vi "PXIe-7962_FPGA.vi"() -> ()   [LabVIEW 2014]
uses:
  <instrlib>/_niInstr/Streaming/v1/Common/Stream State.ctl
  <vilib>/Platform/TimedLoop/XDataNode/timing_clust.ctl
  <vilib>/Platform/TimedLoop/XDataNode/nitl_modes.ctl
  <vilib>/Platform/TimedLoop/XDataNode/wakeup.ctl
  FPGA_Controls/Acquisition FIFOs Cluster.ctl
  <vilib>/rvi/Emulation/niFpgaSctlEmulationGetInTimedLoop.vi
  <vilib>/rvi/Emulation/niFpgaEmulationReportErrorSimple.vi
  <vilib>/rvi/Emulation/niFpgaGetClockAttributes.vi
  <vilib>/rvi/Emulation/niFpgaCriticalErrorInLSC.vi
  <vilib>/rvi/eio/common/nirviEmuTemplateMethod_errors.vi
  <vilib>/rvi/interface/RandomDataEmulation/niFpgaRandomDataHandleErrors.vi
  <vilib>/rvi/DataTransferAndStorage/Container/Common/niFpgaContainerExecOnDevCompGetState.vi
  <vilib>/rvi/Emulation/niFpgaEmulationIsFPGAContextNoSignature.vi
  <vilib>/rvi/errors/niFpgaSetErrorForExecOnDevCompSimple.vi
  <vilib>/rvi/eio/common/nirviEmuReportErrorAndStop.vi
  <vilib>/rvi/DataTransferAndStorage/Container/Common/niFpgaContainerGetUniqueNameForEmu.vi
  <vilib>/rvi/FIFO/Fifo_Resource/nirvififoEmulationSetSize.vi
  <vilib>/rvi/FIFO/Fifo_Resource/nirviFifoEmulationQueueMgr.vi
  <instcachedir>/0/nirviFifoEmulationQueueMgr_E5CAEC123FF24DC58D834DCA3CDAA9B5.lvgen/nirviFifoEmulationQueueMgr_E5CAEC123FF24DC58D834DCA3CDAA9B5_004.vi
  <vilib>/rvi/FIFO/Fifo_Resource/nirvififoEmulationDetermineInputValidOut.vi
  <vilib>/rvi/FIFO/Fifo_Resource/nirvififoEmulationCreateLock.vi
  <vilib>/rvi/Emulation/niFpgaProcessEmulError.vi
  <vilib>/rvi/FIFO/Fifo_Resource/nirvififoEmulationObtainLock.vi
  <vilib>/rvi/FIFO/Fifo_Resource/nirvififoEmulationReleaseLock.vi
  <vilib>/rvi/occurrence/nirviWaitOnOccurrenceBase.vi
  <vilib>/rvi/errors/nirviReportUnexpectedCaseInternalError.vi
  <vilib>/rvi/errors/nirviReportUnexpectedCaseInternalError (U32).vi
  <vilib>/Utility/error.llb/Clear Errors.vi
  <instcachedir>/0/nirviFifoEmulationQueueMgr_E5CAEC123FF24DC58D834DCA3CDAA9B5.lvgen/nirviFifoEmulationQueueMgr_E5CAEC123FF24DC58D834DCA3CDAA9B5_003.vi
  <vilib>/Platform/TimedLoop/XDataNode/XDataNode.xnode
  <vilib>/eio/EIONode/EIONode.xnode
  <vilib>/rvi/DataTransferAndStorage/Container/XNode/niFpgaContainer.xnode
  <vilib>/rvi/interface/RandomDataEmulation/nirviRandomDataFpgaReadWriteTemplate.vi
  <vilib>/rvi/FIFO/Fifo_Resource/niFpgaFifoEmulationRefIn.vi
  <vilib>/rvi/FIFO/Fifo_Resource/nirvififoEmulationWrite.vi
  <vilib>/Platform/TimedLoop/XDataNode/XDNodeRunTimeDep.lvlib
  <instrlib>/_niInstr/Streaming/v1/FPGA/niInstr Streaming v1 FPGA.lvlib
  <instrlib>/_niInstr/Streaming/v1/Common/niInstr Streaming v1 Common.lvlib
panel:
  out "Init Done":bool
  in  "stream.num samples 1":u64
  out "stream.state 1":T1
  out "stream.samples transferred 1":u64
  in  "stream.request state 1":T1
  out "stream.metadata 1":u64
  out "stream.metadata 0":u64
  in  "stream.request state 0":T1
  out "stream.samples transferred 0":u64
  out "stream.state 0":T1
  in  "stream.num samples 0":u64
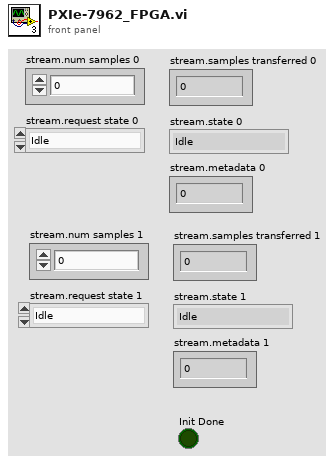
[diagram p1: front panel]
types:
  T1 = typedef "niInstr Streaming v1 Common.lvlib/Stream State.ctl" = enum8{"Idle", "Finite Transfer", "Continuous", "Done", "Error", "Not Ready", "Cancel"}
  T2 = typedef "XDNodeRunTimeDep.lvlib/timing_clust.ctl" = cluster{"Expected End [f-1]":u64, "Actual End [f-1]":u64, "Finished Late? [f-1]":bool, "Expected End [i-1]":u64, "Actual End [i-1]":u64, "Finished Late? [i-1]":bool, "Expected Start [i]":u64, "Actual Start [i]":u64, "Expected Start [f]":u64, "Actual Start [f]":u64, "Source Name":string, "Structure Name":string, "Period":i64, "Deadline":i64, "Offset":i64, "Start":i64, "Priority":i32, "Timeout":i32, "Mode":T3, "Wakeup Reason":T4, "Error":errorcluster, "Source Type":string, "Secondary Source Type":string, "Global End Time":u64, "Global Start Time":u64, "Frame Duration":u64, "Iteration Duration":u64, "Assigned CPU":i32, "I/O Scan Engine Mode":u32}
  T3 = typedef "XDNodeRunTimeDep.lvlib/nitl_modes.ctl" = enum32{"No Change", "Process missed periods, maintain original phase", "Discard missed periods, maintain original phase", "Process missed periods, ignore original phase", "Discard missed periods, ignore original phase"}
  T4 = typedef "XDNodeRunTimeDep.lvlib/wakeup.ctl" = enum32{"Normal", "Aborted", "Asynchronous wakeup", "Timing source error", "Timed loop error", "Timeout"}
  T5 = typedef "Acquisition FIFOs Cluster.ctl" = cluster{"FIFO 0":refnum<k21>, "FIFO 1":refnum<k21>, "FIFO 2":refnum<k21>, "FIFO 3":refnum<k21>, "FIFO 4":refnum<k21>, "FIFO 5":refnum<k21>, "FIFO 6":refnum<k21>, "FIFO 7":refnum<k21>}
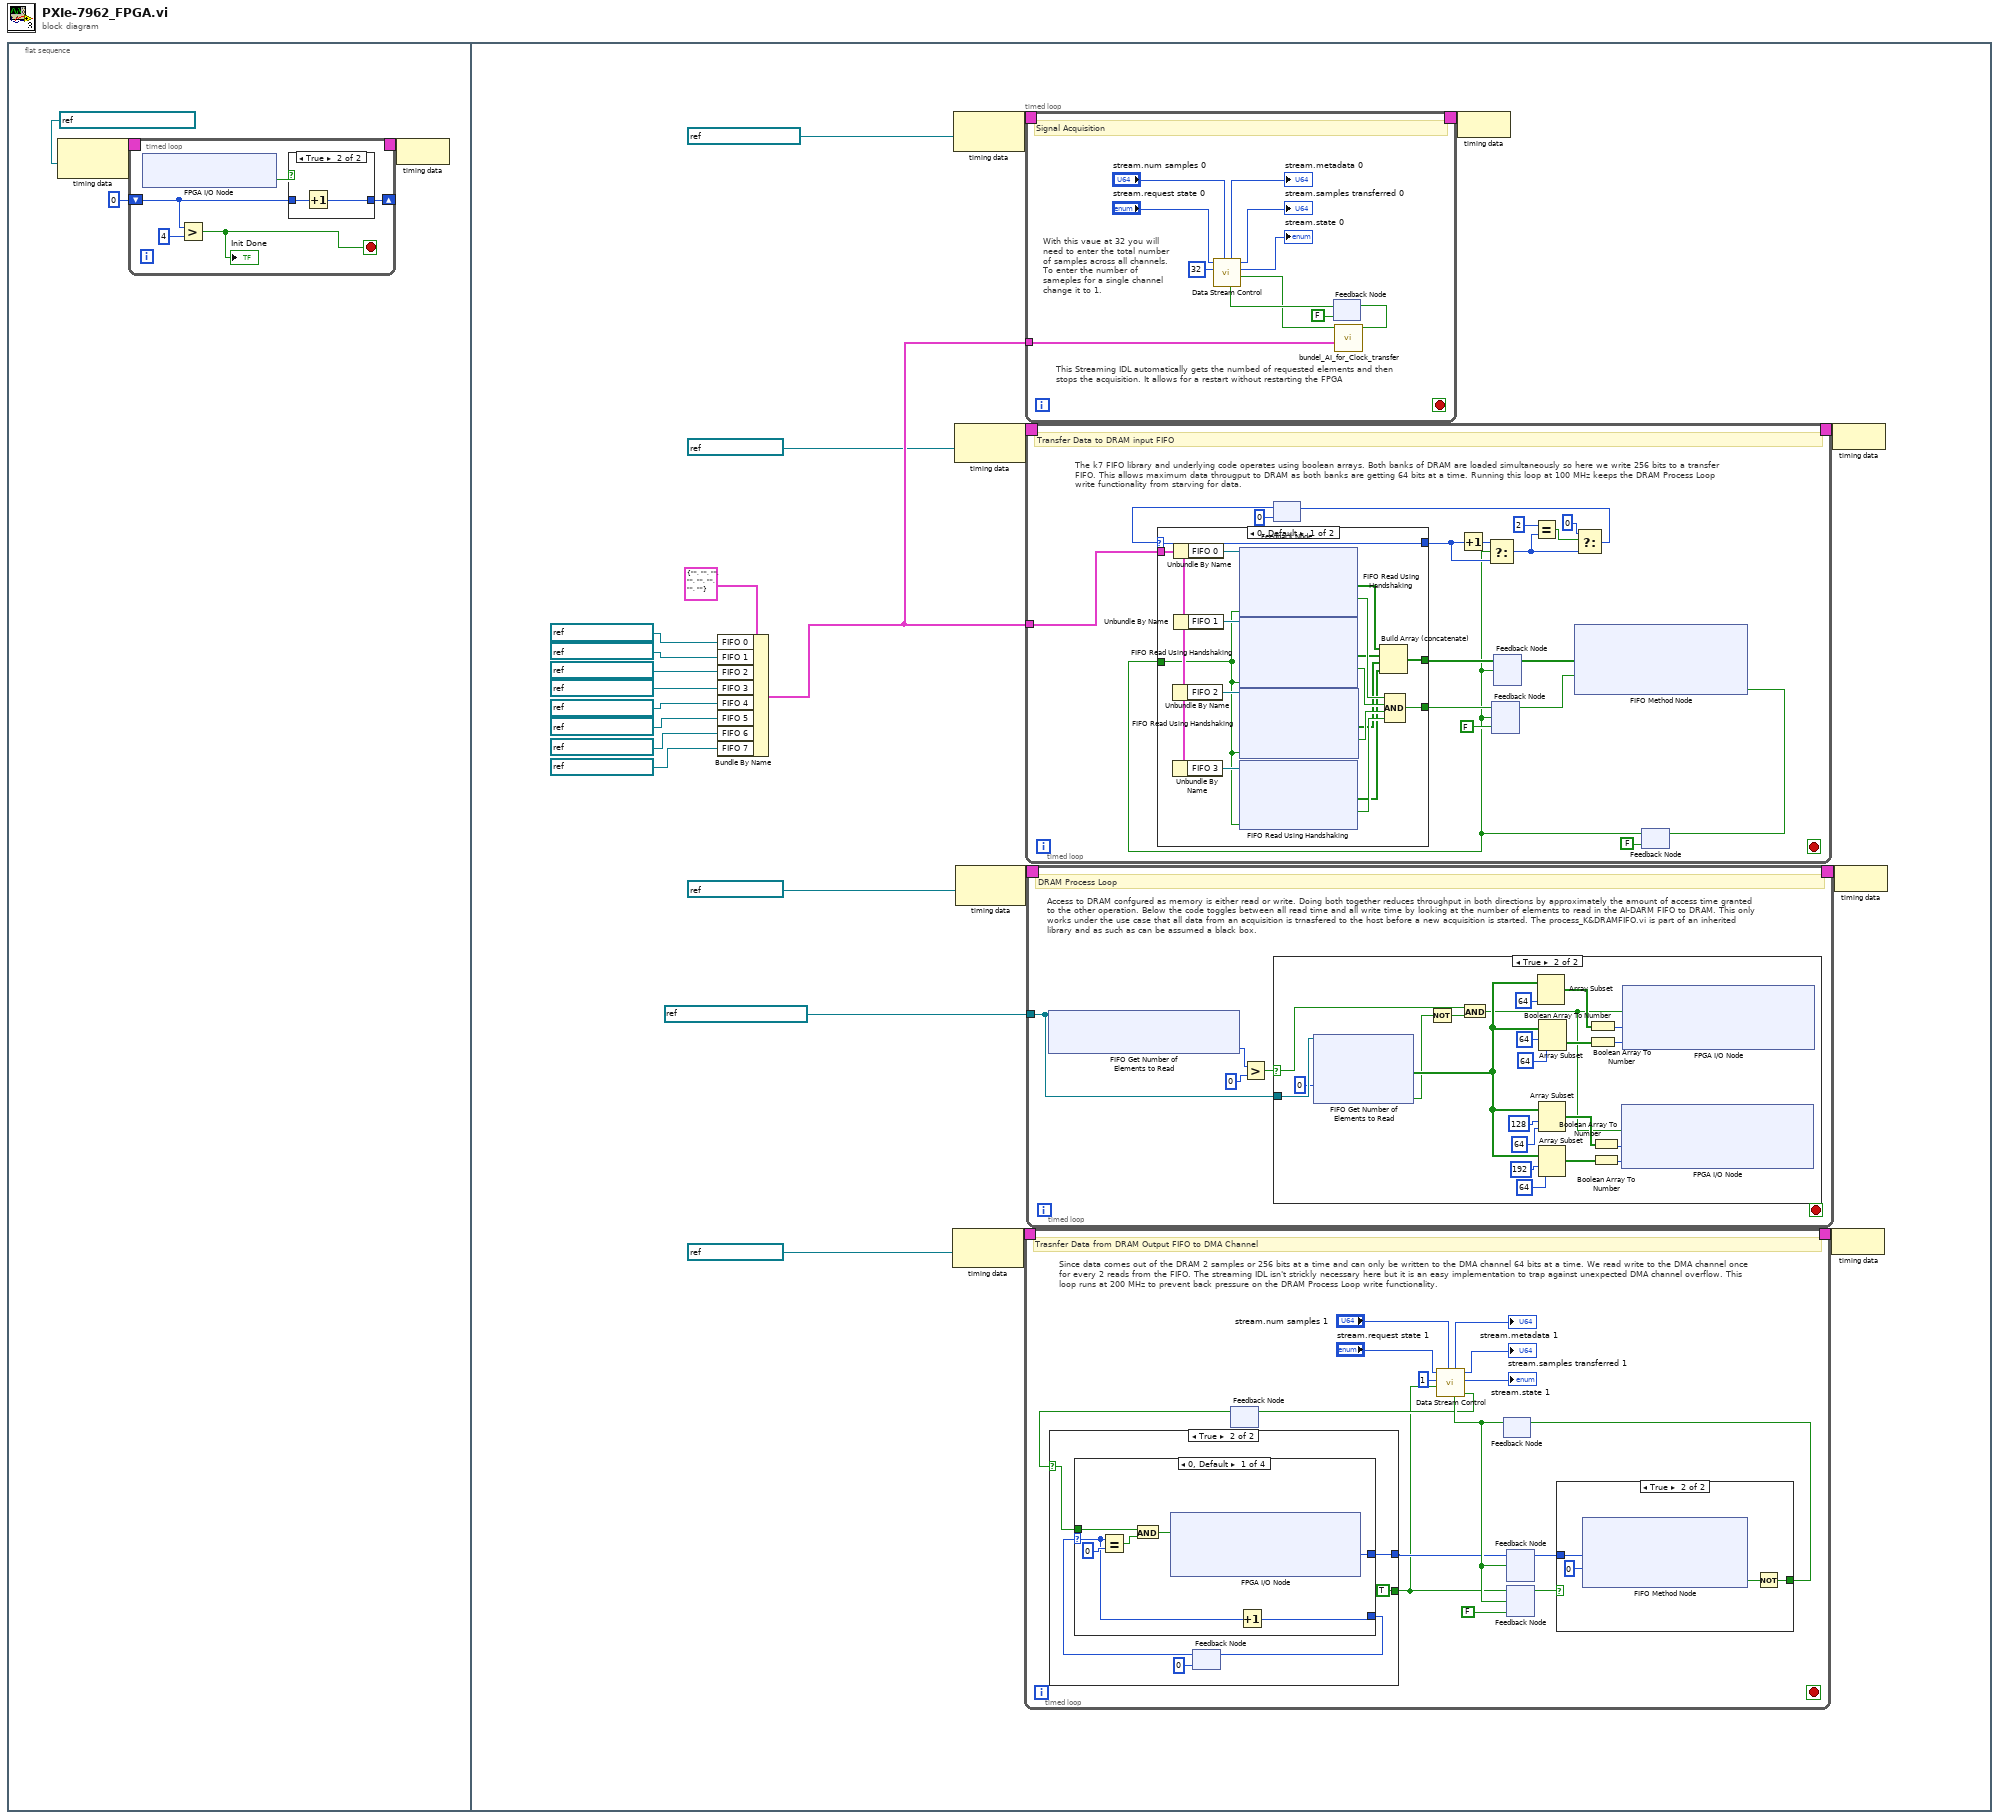
[diagram p0: block diagram]
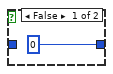
[diagram p2: hidden frame]
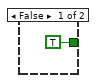
[diagram p3: hidden frame]
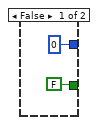
[diagram p4: hidden frame]
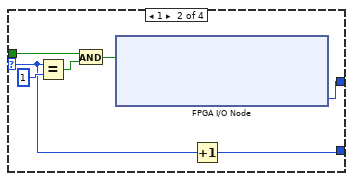
[diagram p5: hidden frame]
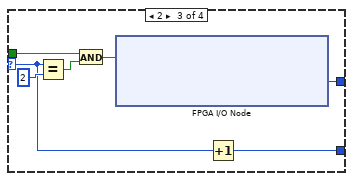
[diagram p6: hidden frame]
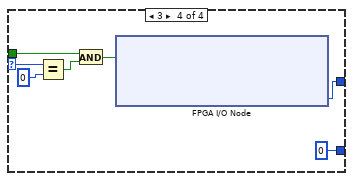
[diagram p7: hidden frame]
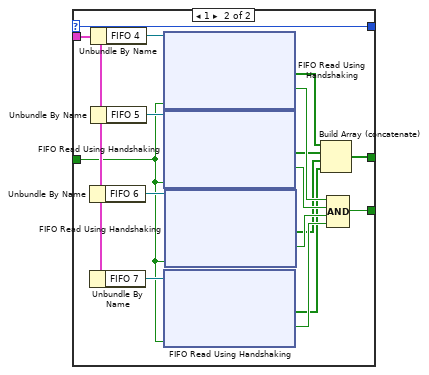
[diagram p9: hidden frame]
diagram:
  n1 = flat-sequence {
    frame #0 {
      n2 = node-c288(refnum<k21> "40 MHz Onboard Clock" ("Source Name")) -> (w4:T2)
      n3 = timed-loop {
        shift-right: [w8] -> _
        shift-left: u16 0 -> [w7]
        timing: w4 -> [_]
        timing-out: [_] -> w3
        stop <- w5 stop-if-true
        n4 = xnode "FPGA I/O Node"() -> ("IO Module\\InitDone"=w9:bool)  [unwired: 1 in, 1 out]
        n5 = Greater?(x=w7, y=u16 4) -> (0:w5:bool)
        "Init Done" <- w5
        n6 = case shown="True" w9 {
          tunnel: [u16 0 w12] -> w8
          tunnel: w7 -> [_ w11]
          frame False {
          }
          frame True {
            n7 = Increment(x=w11) -> (x+1=w12:u16)
          }
        }
      }
      n8 = node-c288(w3) -> ()
    }
    frame #1 {
      n9 = Bundle By Name(cluster=T5 {"FIFO 0"="", "FIFO 1"="", "FIFO 2"="", "FIFO 3"="", "FIFO 4"="", "FIFO 5"="", "FIFO 6"="", "FIFO 7"=""} ("FIFO Refs"), "FIFO 0"=refnum<k21> "AI Bundel FIFO 0" ("FIFO In"), "FIFO 1"=refnum<k21> "AI Bundel FIFO 1" ("FIFO In"), "FIFO 2"=refnum<k21> "AI Bundel FIFO 2" ("FIFO In"), "FIFO 3"=refnum<k21> "AI Bundel FIFO 3" ("FIFO In"), "FIFO 4"=refnum<k21> "AI Bundel FIFO 4" ("FIFO In"), "FIFO 5"=refnum<k21> "AI Bundel FIFO 5" ("FIFO In"), "FIFO 6"=refnum<k21> "AI Bundel FIFO 6" ("FIFO In"), "FIFO 7"=refnum<k21> "AI Bundel FIFO 7" ("FIFO In")) -> (w23:T5)
      n10 = node-c288(refnum<k21> "100 MHz Clock" ("Source Name")) -> (w35:T2)
      n11 = node-c288(refnum<k21> "IO Module Clock 0" ("Source Name")) -> (w41:T2)
      n12 = node-c288(refnum<k21> "100 MHz Clock" ("Source Name")) -> (w39:T2)
      n13 = node-c288(refnum<k21> "100 MHz Clock" ("Source Name")) -> (w37:T2)
      n14 = timed-loop {
        timing: w35 -> [_]
        timing-out: [_] -> w34
        stop <- _ stop-if-true
        # "Since data comes out of the DRAM 2 samples or 256 bits at a time and can only be written to the DMA channel 64 bits at a time. We read write to the DMA channel once for every 2 reads from the FIFO. The streaming IDL isn't strickly necessary here but it is an easy implementation to trap against unexpected DMA channel overflow. This loop runs at 200 MHz to prevent back pressure on the DRAM Process Loop write functionality."
        # "Trasnfer Data from DRAM Output FIFO to DMA Channel"
        n15 = feedback #1() -> (w46:bool)  [unwired: 1 in]
        n16 = case shown="True" w46 {
          selector: w46 -> [_ w69]
          tunnel: [u64 0 ("DRAM Bank 1\\Read_Data_Lower") w68] -> w43
          tunnel: [FALSE TRUE] -> w42
          frame False {
          }
          frame True {
            n17 = feedback #2(i16 0) -> (w65:i16)
            n18 = case shown="0, Default" w65 {
              selector: w65 -> [w71 w77 w84 w92]
              tunnel: w69 -> [w73 w80 w87 w94]
              tunnel: [w72 w79 w86 w93] -> w68
              tunnel: [w70 w78 w85 i16 0] -> w66
              frame 0, Default {
                n19 = Equal?(x=w71, y=i16 0) -> (x = y?=w75:bool)
                n20 = And(x=w73, y=w75) -> (x .and. y?=w74:bool)
                n21 = xnode "FPGA I/O Node"("DRAM Bank 0\\Read"=w74) -> ("DRAM Bank 0\\Read_Data_Upper"=w72:u64)  [unwired: 3 in, 4 out]
                n22 = Increment(x=w71) -> (x+1=w70:i16)
              }
              frame 1 {
                n23 = Equal?(x=w77, y=i16 1) -> (x = y?=w82:bool)
                n24 = And(x=w80, y=w82) -> (x .and. y?=w81:bool)
                n25 = xnode "FPGA I/O Node"("DRAM Bank 0\\Read"=w81) -> ("DRAM Bank 0\\Read_Data_Lower"=w79:u64)  [unwired: 3 in, 4 out]
                n26 = Increment(x=w77) -> (x+1=w78:i16)
              }
              frame 2 {
                n27 = Equal?(x=w84, y=i16 2) -> (x = y?=w89:bool)
                n28 = And(x=w87, y=w89) -> (x .and. y?=w88:bool)
                n29 = xnode "FPGA I/O Node"("DRAM Bank 1\\Read"=w88) -> ("DRAM Bank 1\\Read_Data_Upper"=w86:u64)  [unwired: 3 in, 4 out]
                n30 = Increment(x=w84) -> (x+1=w85:i16)
              }
              frame 3 {
                n31 = Equal?(x=w92, y=i16 0) -> (x = y?=w96:bool)
                n32 = And(x=w94, y=w96) -> (x .and. y?=w95:bool)
                n33 = xnode "FPGA I/O Node"("DRAM Bank 1\\Read"=w95) -> ("DRAM Bank 1\\Read_Data_Lower"=w93:u64)  [unwired: 3 in, 4 out]
              }
            }
            n34 = feedback-in #2(w66) -> ()
          }
        }
        n35 = feedback #3() -> (w48:bool)  [unwired: 1 in]
        n36 = call <instrlib>:"Data Stream Control.vi"("ready for input?"=w48, "stream.num samples 0"="stream.num samples 1", "data valid"=w42, "element count"=u16 1, "stream.request state 0"="stream.request state 1") -> ("request data"=w47:bool, "stream.state 0"=→"stream.state 1":T1, "stream.samples transferred 0"=→"stream.samples transferred 1":u64, "stream.metadata 0"=→"stream.metadata 1":u64)  [unwired: 2 in, 1 out]
        n37 = feedback-in #1(w47) -> ()
        n38 = feedback-in #4(w43, w48) -> ()
        n39 = feedback #4() -> (w56:u64)  [unwired: 1 in]
        n40 = feedback #5(FALSE ("Output Valid")) -> (w44:bool)
        n41 = feedback-in #5(w42, w48) -> ()
        n42 = case shown="True" w44 {
          tunnel: w56 -> [_ w61]
          tunnel: [TRUE w59] -> w45
          frame False {
          }
          frame True {
            n43 = xnode ("FIFO Method Node")("Element"=w61, "Timeout"=0) -> ("Timed Out?"=w60:bool)  [unwired: 1 in, 1 out]
            n44 = Not(x=w60) -> (.not. x?=w59:bool)
          }
        }
        n45 = feedback-in #3(w45) -> ()
      }
      n46 = timed-loop {
        timing: w41 -> [_]
        timing-out: [_] -> w40
        tunnel: w23 -> [w194]
        stop <- _ stop-if-true
        # "With this vaue at 32 you will need to enter the total number of samples across all channels. To enter the number of sameples for a single channel change it to 1."
        # "This Streaming IDL automatically gets the numbed of requested elements and then stops the acquisition. It allows for a restart without restarting the FPGA"
        # "Signal Acquisition"
        n47 = feedback #6(FALSE ("Ready for Input")) -> (w196:bool)
        n48 = call <instrlib>:"Data Stream Control.vi"("ready for input?"=w196, "stream.num samples 0"="stream.num samples 0", "element count"=u16 32, "stream.request state 0"="stream.request state 0") -> ("send data"=w195:bool, "stream.state 0"=→"stream.state 0":T1, "stream.samples transferred 0"=→"stream.samples transferred 0":u64, "stream.metadata 0"=→"stream.metadata 0":u64)  [unwired: 3 in, 1 out]
        n49 = call "bundel_AI_for_Clock_transfer.vi"("FIFO Refs"=w194, "Input Valid"=w195) -> ("Ready for Input"=w204:bool)  [unwired: 9 in]
        n50 = feedback-in #6(w204) -> ()
      }
      n51 = timed-loop {
        timing: w39 -> [_]
        timing-out: [_] -> w38
        tunnel: w23 -> [w153]
        stop <- _ stop-if-true
        # "The k7 FIFO library and underlying code operates using boolean arrays. Both banks of DRAM are loaded simultaneously so here we write 256 bits to a transfer FIFO. This allows maximum data througput to DRAM as both banks are getting 64 bits at a time. Running this loop at 100 MHz keeps the DRAM Process Loop write functionality from starving for data."
        # "Transfer Data to DRAM input FIFO"
        n52 = feedback #7(i16 0 ("t")) -> (w152:i16)
        n53 = feedback #8(FALSE ("Output Valid")) -> (w139:bool)
        n54 = feedback #9() -> (w137:bool[])  [unwired: 1 in]
        n55 = xnode ("FIFO Method Node")("Element"=w137, "Input Valid"=w139) -> ("Ready for Input"=w138:bool)  [unwired: 1 in, 1 out]
        n56 = feedback-in #10(w138) -> ()
        n57 = feedback #10(FALSE ("Ready for Input")) -> (w136:bool)
        n58 = case shown="0, Default" w152 {
          selector: w152 -> [w169 w186]
          tunnel: w153 -> [w155 w172]
          tunnel: [w167 w184] -> w140
          tunnel: [w160 w177] -> w151
          tunnel: [w169 w186] -> w147
          tunnel: w136 -> [w154 w171]
          frame 0, Default {
            n59 = Unbundle By Name(w155) -> ("FIFO 2"=w166:refnum<k21>)
            n60 = Unbundle By Name(w155) -> ("FIFO 3"=w165:refnum<k21>)
            n61 = Unbundle By Name(w155) -> ("FIFO 0"=w170:refnum<k21>)
            n62 = Unbundle By Name(w155) -> ("FIFO 1"=w168:refnum<k21>)
            n63 = xnode ("FIFO Read Using Handshaking")("Ready for Output"=w154, "FIFO In"=w170) -> ("Element"=w159:bool[], "Output Valid"=w164:bool)  [unwired: 1 out]
            n64 = xnode ("FIFO Read Using Handshaking")("Ready for Output"=w154, "FIFO In"=w168) -> ("Element"=w158:bool[], "Output Valid"=w163:bool)  [unwired: 1 out]
            n65 = xnode ("FIFO Read Using Handshaking")("Ready for Output"=w154, "FIFO In"=w165) -> ("Element"=w156:bool[], "Output Valid"=w161:bool)  [unwired: 1 out]
            n66 = xnode ("FIFO Read Using Handshaking")("Ready for Output"=w154, "FIFO In"=w166) -> ("Element"=w157:bool[], "Output Valid"=w162:bool)  [unwired: 1 out]
            n67 = Build Array (concatenate)(w159, w158, w157, w156) -> (w167:bool[])
            n68 = Compound Arithmetic op=AND(w164, w163, w162, w161) -> (w160:bool)
          }
          frame 1 {
            n69 = Unbundle By Name(w172) -> ("FIFO 6"=w183:refnum<k21>)
            n70 = Unbundle By Name(w172) -> ("FIFO 7"=w182:refnum<k21>)
            n71 = Unbundle By Name(w172) -> ("FIFO 4"=w187:refnum<k21>)
            n72 = Unbundle By Name(w172) -> ("FIFO 5"=w185:refnum<k21>)
            n73 = xnode ("FIFO Read Using Handshaking")("Ready for Output"=w171, "FIFO In"=w187) -> ("Element"=w176:bool[], "Output Valid"=w181:bool)  [unwired: 1 out]
            n74 = xnode ("FIFO Read Using Handshaking")("Ready for Output"=w171, "FIFO In"=w185) -> ("Element"=w175:bool[], "Output Valid"=w180:bool)  [unwired: 1 out]
            n75 = xnode ("FIFO Read Using Handshaking")("Ready for Output"=w171, "FIFO In"=w182) -> ("Element"=w173:bool[], "Output Valid"=w178:bool)  [unwired: 1 out]
            n76 = xnode ("FIFO Read Using Handshaking")("Ready for Output"=w171, "FIFO In"=w183) -> ("Element"=w174:bool[], "Output Valid"=w179:bool)  [unwired: 1 out]
            n77 = Build Array (concatenate)(w176, w175, w174, w173) -> (w184:bool[])
            n78 = Compound Arithmetic op=AND(w181, w180, w179, w178) -> (w177:bool)
          }
        }
        n79 = Increment(x=w147) -> (x+1=w148:i16)
        n80 = Select(t=w148, s=w136, f=w147) -> (s? t:f=w145:i16)
        n81 = feedback-in #8(w151, w136) -> ()
        n82 = feedback-in #9(w140, w136) -> ()
        n83 = Equal?(x=i16 2, y=w145) -> (x = y?=w144:bool)
        n84 = Select(t=i16 0, s=w144, f=w145) -> (s? t:f=w143:i16)
        n85 = feedback-in #7(w143) -> ()
      }
      n86 = timed-loop {
        timing: w37 -> [_]
        timing-out: [_] -> w36
        tunnel: refnum<k21> "Bundeling to DRAM FIFO" ("FIFO In") -> [w104]
        stop <- _ stop-if-true
        # "Access to DRAM confgured as memory is either read or write. Doing both together reduces throughput in both directions by approximately the amount of access time granted to the other operation. Below the code toggles between all read time and all write time by looking at the number of elements to read in the AI-DARM FIFO to DRAM. This only works under the use case that all data from an acquisition is trnasfered to the host before a new acquisition is started. The process_K&DRAMFIFO.vi is part of an inherited library and as such as can be assumed a black box."
        # "DRAM Process Loop"
        n87 = xnode ("FIFO Get Number of Elements to Read")("FIFO In"=w104) -> ("Number of Elements to Read"=w107:u32)  [unwired: 1 out]
        n88 = Greater?(x=w107, y=u32 0) -> (0:w105:bool)
        n89 = case shown="True" w105 {
          selector: w105 -> [_ w112]
          tunnel: w104 -> [_ w129]
          frame False {
          }
          frame True {
            n90 = xnode ("FIFO Get Number of Elements to Read")("Timeout"=0, "FIFO In"=w129) -> ("Element"=w118:bool[], "Timed Out?"=w110:bool)  [unwired: 1 out]
            n91 = Not(x=w110) -> (.not. x?=w111:bool)
            n92 = And(x=w112, y=w111) -> (x .and. y?=w109:bool)
            n93 = Array Subset(array=w118, length=64) -> (w122:bool[])  [unwired: 1 in]
            n94 = Array Subset(array=w118, index=128, length=64) -> (w113:bool[])
            n95 = Array Subset(array=w118, index=192, length=64) -> (w114:bool[])
            n96 = Array Subset(array=w118, index=64, length=64) -> (w125:bool[])
            n97 = Boolean Array To Number(Boolean array=w122) -> (number=w123:u64)
            n98 = Boolean Array To Number(Boolean array=w125) -> (number=w124:u64)
            n99 = Boolean Array To Number(Boolean array=w113) -> (number=w116:u64)
            n100 = Boolean Array To Number(Boolean array=w114) -> (number=w115:u64)
            n101 = xnode "FPGA I/O Node"("DRAM Bank 1\\Write"=w109, "DRAM Bank 1\\Write_Data_Upper"=w116, "DRAM Bank 1\\Write_Data_Lower"=w115) -> ()  [unwired: 3 in, 3 out]
            n102 = xnode "FPGA I/O Node"("DRAM Bank 0\\Write"=w109, "DRAM Bank 0\\Write_Data_Upper"=w123, "DRAM Bank 0\\Write_Data_Lower"=w124) -> ()  [unwired: 3 in, 3 out]
          }
        }
      }
      n103 = node-c288(w40) -> ()
      n104 = node-c288(w34) -> ()
      n105 = node-c288(w38) -> ()
      n106 = node-c288(w36) -> ()
    }
  }
